vi "报告打印.vi"(9 "输出簇":T1, 11 "打印?":bool) -> ()   [LabVIEW 2010]
uses:
  <vilib>/Utility/NIReport.llb/NI_report.lvclass
  <vilib>/Utility/NIReport.llb/Append Report Text (str wrap).vi
  全局量/试验配置信息.vi
  <vilib>/addons/_office/word.llb/Word Easy Table (str).vi
  <vilib>/addons/_office/NI_ReportGenerationToolkit.lvlib
  全局量/全局_配置.vi
panel:
  in  "序号":i32
  out "XY图":cluster{"Y":dbl[], "Y":dbl[]}[](graph)
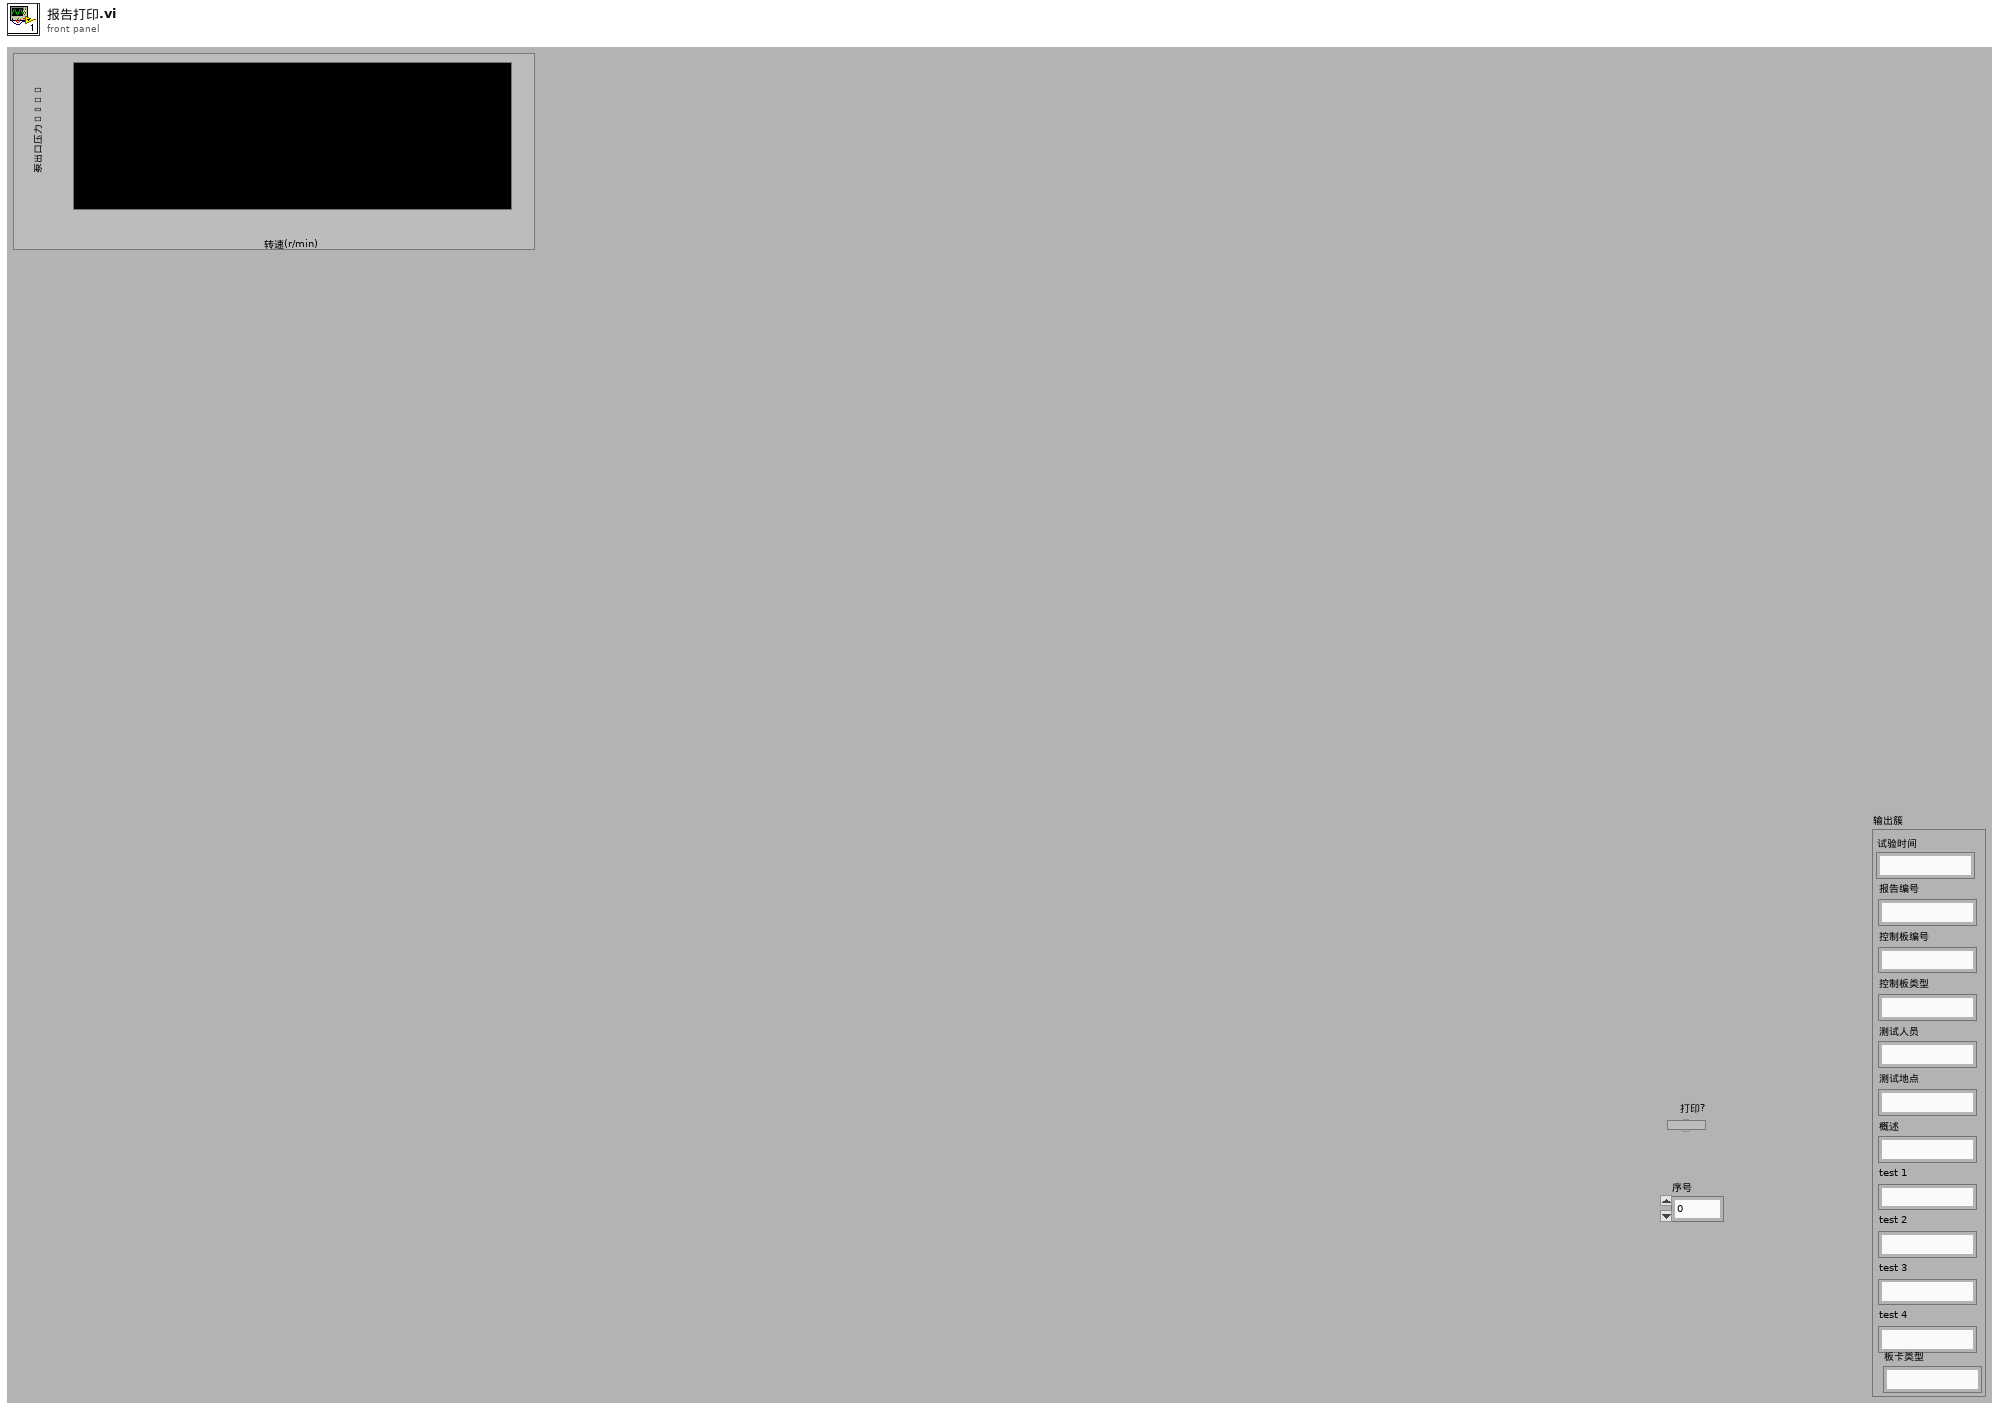
[diagram p1: front panel]
types:
  T1 = cluster{"试验时间":string, "报告编号":string, "控制板编号":string, "控制板类型":string, "测试人员":string, "测试地点":string, "概述":string, "test 1":string, "test 2":string, "test 3":string, "test 4":string, "板卡类型":string}
  T2 = cluster{"position (Excel)":cluster{"row":i32, "column":i32}, "name (Excel)":string, "bookmark (Word)":string}
  T3 = enum16{"maximized", "minimized", "normal", "no change"}
  T4 = enum16{"Standard Report", "HTML", "Word", "Excel"}
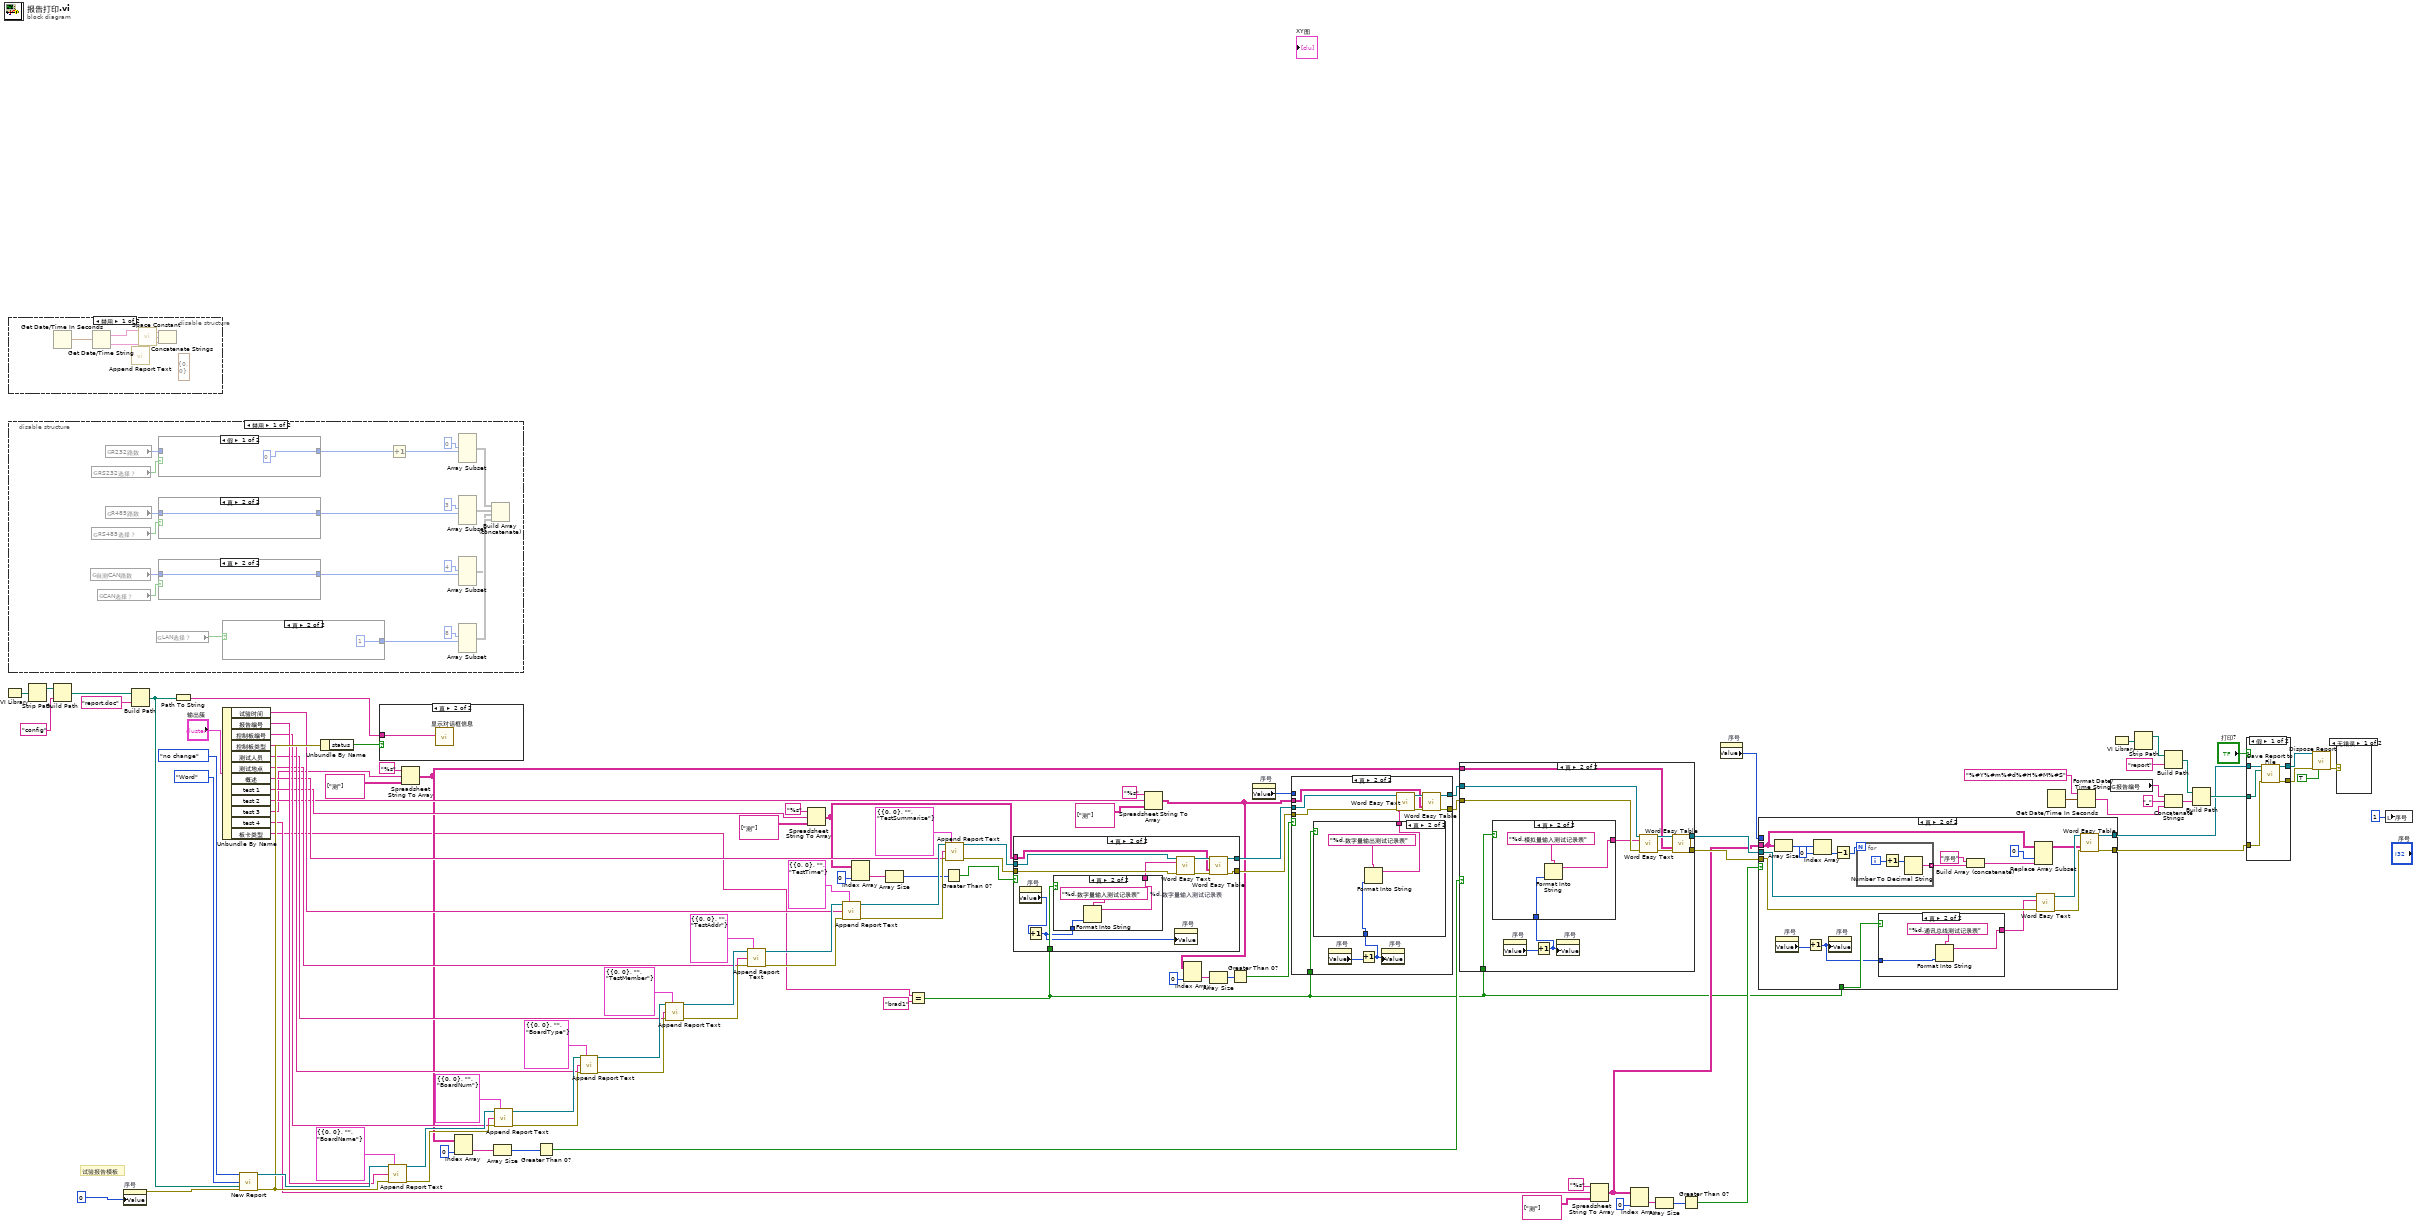
[diagram p0: block diagram]
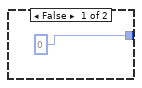
[diagram p2: hidden frame]
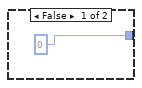
[diagram p3: hidden frame]
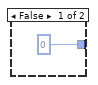
[diagram p5: hidden frame]
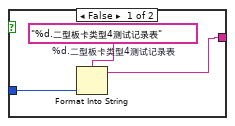
[diagram p8: hidden frame]
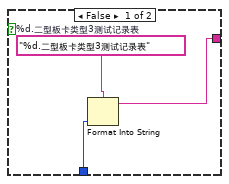
[diagram p10: hidden frame]
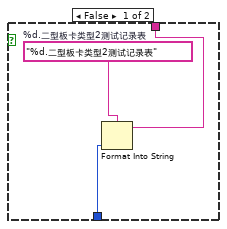
[diagram p12: hidden frame]
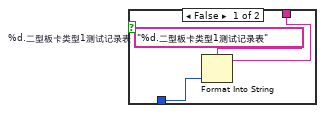
[diagram p14: hidden frame]
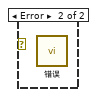
[diagram p15: hidden frame]
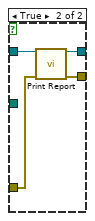
[diagram p16: hidden frame]
diagram:
  # "试验报告模板"
  n1 = VI Library() -> (path=w99:path)
  n2 = disable-structure shown="禁用" {
    frame Disabled {
      (unwired) cluster{"row":i32, "column":i32} {"row"=0, "column"=0} ("position (excel)")
      n3 = Get Date/Time In Seconds() -> (seconds since 1Jan1904=w109:timestamp)
      n4 = Get Date/Time String(seconds (now)=w109) -> (date string=w108:string, time string=w107:string)  [unwired: 2 in]
      n5 = call-poly <vilib>:"Append Report Text.vi"() -> ()  [unwired: 12 in, 4 out]
      n6 = call <vilib>:"Space Constant.vi"() -> ("String"=w106:string)
      n7 = Concatenate Strings(w108, w106, w107) -> ()  [unwired: 1 out]
    }
    frame Enabled {
    }
  }
  n8 = disable-structure shown="禁用" {
    frame Disabled {
      n9 = global read "试验配置信息.vi" "自测CAN路数"() -> (w118:i32)
      n10 = global read "试验配置信息.vi" "RS232选择？"() -> (w124:bool)
      n11 = global read "试验配置信息.vi" "RS485选择？"() -> (w121:bool)
      n12 = global read "试验配置信息.vi" "CAN选择？"() -> (w119:bool)
      n13 = global read "全局_配置.vi" "R232路数"() -> (w123:u32)
      n14 = global read "全局_配置.vi" "R485路数"() -> (w120:u32)
      n15 = global read "试验配置信息.vi" "LAN选择？"() -> (w117:bool)
      n16 = case shown="假" w124 {
        tunnel: w123 -> [_ w135]
        tunnel: [u32 0 ("R232路数") w135] -> w116
        frame False {
        }
        frame True {
        }
      }
      n17 = case shown="真" w121 {
        tunnel: w120 -> [_ w133]
        tunnel: [u32 0 ("R232路数") w133] -> w114
        frame False {
        }
        frame True {
        }
      }
      n18 = case shown="真" w119 {
        tunnel: w118 -> [_ w131]
        tunnel: [u32 0 ("R232路数") w131] -> w112
        frame False {
        }
        frame True {
        }
      }
      n19 = case shown="真" w117 {
        tunnel: [u32 0 ("R232路数") u32 1 ("R232路数")] -> w110
        frame False {
        }
        frame True {
        }
      }
      n20 = Increment(x=w116) -> (x+1=w122:u32)
      n21 = Array Subset(index (row)=0 ("索引"), length (row)=w122) -> (w126:void[][])  [unwired: 3 in]
      n22 = Array Subset(index (row)=3 ("索引"), length (row)=w114) -> (w127:void[][])  [unwired: 3 in]
      n23 = Array Subset(index (row)=4 ("索引"), length (row)=w112) -> (w128:void[][])  [unwired: 3 in]
      n24 = Array Subset(index (row)=8 ("索引"), length (row)=w110) -> (w129:void[][])  [unwired: 3 in]
      n25 = Build Array (concatenate)(w126, w127, w128, w129) -> ()  [unwired: 1 out]
    }
    frame Enabled {
    }
  }
  n26 = Strip Path(path=w99) -> (stripped path=w96:path)  [unwired: 1 out]
  n27 = Build Path(base path=w96, name or relative path="config") -> (appended path=w98:path)
  n28 = property on="序号" class="DigNum (严格)"("Value"=0 ("序号")) -> (error out=w51:errorcluster)  [unwired: 2 in, 1 out]
  n29 = Build Path(base path=w98, name or relative path="report.doc") -> (appended path=w102:path)
  n30 = Path To String(path=w102) -> (string=w103:string)
  n31 = Unbundle By Name("输出簇") -> ("试验时间"=w41:string, "报告编号"=w46:string, "控制板编号"=w45:string, "控制板类型"=w44:string, "测试人员"=w43:string, "测试地点"=w42:string, "概述"=w40:string, "test 1"=w37:string, "test 2"=w27:string, "test 3"=w20:string, "test 4"=w13:string, "板卡类型"=w3:string)
  n32 = call <vilib>:"New Report.vi"("window state (normal)"=T3."no change", "report type"=T4."Word", "template (empty)"=w102, "error in (no error)"=w51) -> ("report out"=w93:refnum<class "NI_report.lvclass">, "error out"=w92:errorcluster)  [unwired: 10 in]
  n33 = Unbundle By Name(w92) -> ("status"=w104:bool)
  n34 = case shown="真" w104 {
    tunnel: w103 -> [_ w138]
    frame False {
    }
    frame True {
      n35 = call "显示对话框信息"("Message"=w138) -> ()  [unwired: 9 in, 2 out]
    }
  }
  n36 = call-poly <vilib>:"Append Report Text.vi"("report in"=w93, "MS Office parameters"=T2 {"position (Excel)"={"row"=0, "column"=0}, "name (Excel)"="", "bookmark (Word)"="BoardName"}, "text"=w46, "error in (no error)"=w92) -> ("report out"=w78:refnum<class "NI_report.lvclass">, "error out"=w77:errorcluster)  [unwired: 8 in, 2 out]
  n37 = Spreadsheet String To Array(format string="%s" ("格式字符串"), spreadsheet string=w20, array type (2D Dbl)=string[][] [["测"]] ("数组类型(2D String)")) -> (array=w18:string[][])  [unwired: 1 in]
  n38 = Index Array(array=w18, index (col)=0 ("禁用的索引 (列)")) -> (element=w21:string[])  [unwired: 1 in]
  n39 = Array Size(array=w21) -> (size(s)=w8:i32)
  n40 = call-poly <vilib>:"Append Report Text.vi"("report in"=w78, "MS Office parameters"=T2 {"position (Excel)"={"row"=0, "column"=0}, "name (Excel)"="", "bookmark (Word)"="BoardNum"}, "text"=w45, "error in (no error)"=w77) -> ("report out"=w88:refnum<class "NI_report.lvclass">, "error out"=w87:errorcluster)  [unwired: 8 in, 2 out]
  n41 = Greater Than 0?(x=w8) -> (x > 0?=w19:bool)
  n42 = call-poly <vilib>:"Append Report Text.vi"("report in"=w88, "MS Office parameters"=T2 {"position (Excel)"={"row"=0, "column"=0}, "name (Excel)"="", "bookmark (Word)"="BoardType"}, "text"=w44, "error in (no error)"=w87) -> ("report out"=w85:refnum<class "NI_report.lvclass">, "error out"=w84:errorcluster)  [unwired: 8 in, 2 out]
  n43 = call-poly <vilib>:"Append Report Text.vi"("report in"=w85, "MS Office parameters"=T2 {"position (Excel)"={"row"=0, "column"=0}, "name (Excel)"="", "bookmark (Word)"="TestMember"}, "text"=w43, "error in (no error)"=w84) -> ("report out"=w82:refnum<class "NI_report.lvclass">, "error out"=w81:errorcluster)  [unwired: 8 in, 2 out]
  n44 = call-poly <vilib>:"Append Report Text.vi"("report in"=w82, "MS Office parameters"=T2 {"position (Excel)"={"row"=0, "column"=0}, "name (Excel)"="", "bookmark (Word)"="TestAddr"}, "text"=w42, "error in (no error)"=w81) -> ("report out"=w80:refnum<class "NI_report.lvclass">, "error out"=w79:errorcluster)  [unwired: 8 in, 2 out]
  n45 = Spreadsheet String To Array(format string="%s" ("格式字符串"), spreadsheet string=w37, array type (2D Dbl)=string[][] [["测"]] ("数组类型(2D String)")) -> (array=w36:string[][])  [unwired: 1 in]
  n46 = call-poly <vilib>:"Append Report Text.vi"("report in"=w80, "MS Office parameters"=T2 {"position (Excel)"={"row"=0, "column"=0}, "name (Excel)"="", "bookmark (Word)"="TestTime"}, "text"=w41, "error in (no error)"=w79) -> ("report out"=w56:refnum<class "NI_report.lvclass">, "error out"=w55:errorcluster)  [unwired: 8 in, 2 out]
  n47 = Index Array(array=w36, index (col)=0 ("禁用的索引 (列)")) -> (element=w34:string[])  [unwired: 1 in]
  n48 = Array Size(array=w34) -> (size(s)=w33:i32)
  n49 = Equal?(x=w3, y="brad1") -> (x = y?=w1:bool)
  n50 = Greater Than 0?(x=w33) -> (x > 0?=w32:bool)
  n51 = call-poly <vilib>:"Append Report Text.vi"("report in"=w56, "MS Office parameters"=T2 {"position (Excel)"={"row"=0, "column"=0}, "name (Excel)"="", "bookmark (Word)"="TestSummarize"}, "text"=w40, "error in (no error)"=w55) -> ("report out"=w54:refnum<class "NI_report.lvclass">, "error out"=w53:errorcluster)  [unwired: 8 in, 2 out]
  n52 = case shown="真" w32 {
    tunnel: [w140 w150] -> w63
    tunnel: [w139 w149] -> w61
    tunnel: w54 -> [w140 w147]
    tunnel: w53 -> [w139 w146]
    tunnel: w36 -> [_ w145]
    tunnel: w1 -> [_ w143]
    frame False {
    }
    frame True {
      n53 = property on="序号" class="DigNum (严格)"() -> ("Value"=w141:i32)  [unwired: 2 in, 2 out]
      n54 = Increment(x=w141) -> (x+1=w142:i32)
      n55 = case shown="真" w143 {
        tunnel: [w153 w155] -> w144
        tunnel: w142 -> [w152 w157]
        frame False {
          w154 = "%d.二型板卡类型1测试记录表"  # %d.二型板卡类型1测试记录表
          n56 = Format Into String(format string=w154, w152) -> (resulting string=w153:string)  [unwired: 2 in, 1 out]
        }
        frame True {
          w156 = "%d.数字量输入测试记录表"  # %d.数字量输入测试记录表
          n57 = Format Into String(format string=w156, w157) -> (resulting string=w155:string)  [unwired: 2 in, 1 out]
        }
      }
      n58 = property on="序号" class="DigNum (严格)"("Value"=w142) -> ()  [unwired: 2 in, 2 out]
      n59 = call <vilib>:"Word Easy Text.vi"("report in"=w147, "text"=w144, "error in (no error)"=w146) -> ("report out"=w151:refnum<class "NI_report.lvclass">, "error out"=w148:errorcluster)  [unwired: 10 in, 1 out]
      n60 = call-poly <vilib>:"Word Easy Table.vi"("report in"=w151, "data"=w145, "error in (no error)"=w148) -> ("report out"=w150:refnum<class "NI_report.lvclass">, "error out"=w149:errorcluster)  [unwired: 10 in, 1 out]
    }
  }
  n61 = Spreadsheet String To Array(format string="%s" ("格式字符串"), spreadsheet string=w27, array type (2D Dbl)=string[][] [["测"]] ("数组类型(2D String)")) -> (array=w25:string[][])  [unwired: 1 in]
  n62 = Index Array(array=w25, index (col)=0 ("禁用的索引 (列)")) -> (element=w28:string[])  [unwired: 1 in]
  n63 = Array Size(array=w28) -> (size(s)=w9:i32)
  n64 = Greater Than 0?(x=w9) -> (x > 0?=w26:bool)
  n65 = property on="序号" class="DigNum (严格)"() -> ("Value"=w10:i32)  [unwired: 2 in, 2 out]
  n66 = case shown="真" w26 {
    tunnel: w63 -> [w159 w170]
    tunnel: [w159 w168] -> w62
    tunnel: w61 -> [w158 w167]
    tunnel: [w158 w165] -> w60
    tunnel: w10 -> [_ _]
    tunnel: w25 -> [_ w164]
    tunnel: w1 -> [_ w162]
    frame False {
    }
    frame True {
      n67 = property on="序号" class="DigNum (严格)"() -> ("Value"=w161:i32)  [unwired: 2 in, 2 out]
      n68 = Increment(x=w161) -> (x+1=w160:i32)
      n69 = case shown="真" w162 {
        tunnel: [w173 w175] -> w163
        tunnel: w160 -> [w171 w174]
        frame False {
          w172 = "%d.二型板卡类型2测试记录表"  # %d.二型板卡类型2测试记录表
          n70 = Format Into String(format string=w172, w171) -> (resulting string=w173:string)  [unwired: 2 in, 1 out]
        }
        frame True {
          n71 = Format Into String(format string="%d.数字量输出测试记录表", w174) -> (resulting string=w175:string)  [unwired: 2 in, 1 out]
        }
      }
      n72 = property on="序号" class="DigNum (严格)"("Value"=w160) -> ()  [unwired: 2 in, 2 out]
      n73 = call <vilib>:"Word Easy Text.vi"("report in"=w170, "text"=w163, "error in (no error)"=w167) -> ("report out"=w169:refnum<class "NI_report.lvclass">, "error out"=w166:errorcluster)  [unwired: 10 in, 1 out]
      n74 = call-poly <vilib>:"Word Easy Table.vi"("report in"=w169, "data"=w164, "error in (no error)"=w166) -> ("report out"=w168:refnum<class "NI_report.lvclass">, "error out"=w165:errorcluster)  [unwired: 10 in, 1 out]
    }
  }
  n75 = case shown="真" w19 {
    tunnel: w62 -> [w178 w189]
    tunnel: w60 -> [w177 w187]
    tunnel: [w178 w185] -> w59
    tunnel: [w177 w184] -> w58
    tunnel: w18 -> [_ w183]
    tunnel: w1 -> [_ w181]
    frame False {
    }
    frame True {
      n76 = property on="序号" class="DigNum (严格)"() -> ("Value"=w180:i32)  [unwired: 2 in, 2 out]
      n77 = Increment(x=w180) -> (x+1=w179:i32)
      n78 = case shown="真" w181 {
        tunnel: [w191 w193] -> w182
        tunnel: w179 -> [w190 w195]
        frame False {
          w192 = "%d.二型板卡类型3测试记录表"  # %d.二型板卡类型3测试记录表
          n79 = Format Into String(format string=w192, w190) -> (resulting string=w191:string)  [unwired: 2 in, 1 out]
        }
        frame True {
          n80 = Format Into String(format string="%d.模拟量输入测试记录表", w195) -> (resulting string=w193:string)  [unwired: 2 in, 1 out]
        }
      }
      n81 = property on="序号" class="DigNum (严格)"("Value"=w179) -> ()  [unwired: 2 in, 2 out]
      n82 = call <vilib>:"Word Easy Text.vi"("report in"=w189, "text"=w182, "error in (no error)"=w187) -> ("report out"=w188:refnum<class "NI_report.lvclass">, "error out"=w186:errorcluster)  [unwired: 10 in, 1 out]
      n83 = call-poly <vilib>:"Word Easy Table.vi"("report in"=w188, "data"=w183, "error in (no error)"=w186) -> ("report out"=w185:refnum<class "NI_report.lvclass">, "error out"=w184:errorcluster)  [unwired: 10 in, 1 out]
    }
  }
  n84 = Spreadsheet String To Array(format string="%s" ("格式字符串"), spreadsheet string=w13, array type (2D Dbl)=string[][] [["测"]] ("数组类型(2D String)")) -> (array=w11:string[][])  [unwired: 1 in]
  n85 = Index Array(array=w11, index (col)=0 ("禁用的索引 (列)")) -> (element=w14:string[])  [unwired: 1 in]
  n86 = Array Size(array=w14) -> (size(s)=w6:i32)
  n87 = Greater Than 0?(x=w6) -> (x > 0?=w12:bool)
  n88 = property on="序号" class="DigNum (严格)"() -> ("Value"=w7:i32)  [unwired: 2 in, 2 out]
  n89 = case shown="真" w12 {
    tunnel: [w197 w217] -> w65
    tunnel: [w196 w216] -> w64
    tunnel: w59 -> [w197 w215]
    tunnel: w58 -> [w196 w214]
    tunnel: w7 -> [_ _]
    tunnel: w11 -> [_ w206]
    tunnel: w1 -> [_ w200]
    frame False {
    }
    frame True {
      n90 = Array Size(array=w206) -> (size(s)=w210:i32[])
      n91 = property on="序号" class="DigNum (严格)"() -> ("Value"=w199:i32)  [unwired: 2 in, 2 out]
      n92 = Increment(x=w199) -> (x+1=w198:i32)
      n93 = Index Array(array=w210, index=0 ("索引")) -> (element=w205:i32)
      n94 = property on="序号" class="DigNum (严格)"("Value"=w198) -> ()  [unwired: 2 in, 2 out]
      n95 = Decrement(x=w205) -> (x-1=w204:i32)
      n96 = for {
        N: w204 -> [_]
        tunnel: [w224] -> w202 mode=indexing
        i -> [w226]
        n97 = Increment(x=w226) -> (x+1=w225:i32)
        n98 = Number To Decimal String(number=w225) -> (decimal integer string=w224:string)  [unwired: 1 in]
      }
      n99 = case shown="真" w200 {
        tunnel: [w220 w221] -> w211
        tunnel: w198 -> [w218 w223]
        frame False {
          w219 = "%d.二型板卡类型4测试记录表"  # %d.二型板卡类型4测试记录表
          n100 = Format Into String(format string=w219, w218) -> (resulting string=w220:string)  [unwired: 2 in, 1 out]
        }
        frame True {
          n101 = Format Into String(format string="%d.通讯总线测试记录表", w223) -> (resulting string=w221:string)  [unwired: 2 in, 1 out]
        }
      }
      n102 = Build Array (concatenate)("序号", w202) -> (w201:string[])
      n103 = Replace Array Subset(array=w206, new element=w201, index (col)=0 ("索引 (行)")) -> (w207:string[][])  [unwired: 1 in]
      n104 = call <vilib>:"Word Easy Text.vi"("report in"=w215, "text"=w211, "error in (no error)"=w214) -> ("report out"=w213:refnum<class "NI_report.lvclass">, "error out"=w212:errorcluster)  [unwired: 10 in, 1 out]
      n105 = call-poly <vilib>:"Word Easy Table.vi"("report in"=w213, "data"=w207, "error in (no error)"=w212) -> ("report out"=w217:refnum<class "NI_report.lvclass">, "error out"=w216:errorcluster)  [unwired: 10 in, 1 out]
    }
  }
  n106 = Get Date/Time In Seconds() -> (seconds since 1Jan1904=w71:timestamp)
  n107 = Format Date/Time String(time format string (%c)="%#Y%#m%#d%#H%#M%#S" ("时间格式字符串(%c)"), seconds (now)=w71) -> (date/time string=w50:string)  [unwired: 1 in]
  n108 = global read "试验配置信息.vi" "报告编号"() -> (w49:string)
  n109 = VI Library() -> (path=w72:path)
  n110 = Strip Path(path=w72) -> (stripped path=w75:path)  [unwired: 1 out]
  n111 = Build Path(base path=w75, name or relative path="report") -> (appended path=w73:path)
  n112 = Concatenate Strings(w49, "_", w50) -> (w47:string)
  n113 = Build Path(base path=w73, name or relative path=w47) -> (appended path=w67:path)
  n114 = case shown="假" "打印?" {
    tunnel: w65 -> [w231 w235]
    tunnel: w64 -> [w230 w234]
    tunnel: [w229 w233] -> w69
    tunnel: [w228 w232] -> w68
    tunnel: w67 -> [w227 _]
    frame False {
      n115 = call-dynamic "Save Report to File.vi"("report in"=w231, "report file path"=w227, "error in (no error)"=w230) -> ("report out"=w229:refnum<class "NI_report.lvclass">, "error out"=w228:errorcluster)  [unwired: 11 in]
    }
    frame True {
      n116 = call-dynamic "Print Report.vi"("report in"=w235, "error in (no error)"=w234) -> ("report out"=w233:refnum<class "NI_report.lvclass">, "error out"=w232:errorcluster)  [unwired: 12 in]
    }
  }
  n117 = call-dynamic "Dispose Report.vi"("report in"=w69, "error in (no error)"=w68, "close report? (T)"=TRUE) -> ("error out"=w66:errorcluster)  [unwired: 12 in]
  n118 = case shown="无错误" w66 {
    frame No Error {
    }
    frame Error {
      n119 = call "错误"() -> ()  [unwired: 10 in, 2 out]
    }
  }
  n120 = local write "序号"(1) -> ()
